vi "_System Polling.vi"   [LabVIEW 2012]
uses:
  <vilib>/rvi/DataTransferAndStorage/Container/Common/niFpgaContainerGetUniqueNameForEmu.vi
  <vilib>/rvi/Memory/Memory_Emulation/niFpgaMemoryEmulationCacheClearOnFirstRun.vi
  <vilib>/rvi/Memory/Memory_Emulation/nirvimemoryEmulationManagerCache_MakeExclusive.vi
  <vilib>/rvi/Memory/Memory_Emulation/niFpgaMemoryEmulationValidateCache.vi
  <vilib>/rvi/Memory/Memory_Emulation/nirvimemoryEmulationManagerCache_ReleaseExclusive.vi
  <vilib>/rvi/Memory/Memory_Emulation/nirvimemoryEmulationManagerCache_InsertValue.vi
  <vilib>/Utility/error.llb/Clear Errors.vi
  <vilib>/rvi/Emulation/niFpgaSctlEmulationGetInTimedLoop.vi
  <vilib>/rvi/Memory/Memory_Emulation/nirvimemoryEmulationManagerCache_GetValue.vi
  <vilib>/rvi/Memory/Memory_Emulation/nirvimemoryEmulationManagerCache_SetValue.vi
  <vilib>/rvi/Emulation/niFpgaSctlEmulationResourceMgr.vi
  <vilib>/rvi/DataTransferAndStorage/Container/XNode/niFpgaContainer.xnode
  <vilib>/rvi/Memory/Memory_Emulation/nirvimemoryEmulation.vi
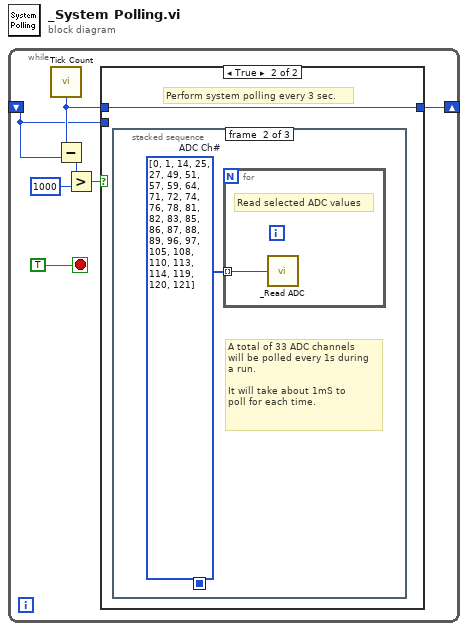
[diagram p0: block diagram]
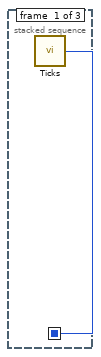
[diagram p3: hidden frame]
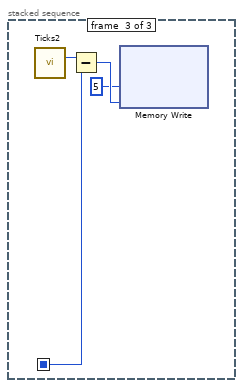
[diagram p4: hidden frame]
diagram:
  n1 = while {
    shift-right: [w1] -> _
    shift-left: _ -> [w2]
    stop <- TRUE stop-if-true
    n2 = call "Tick Count"() -> ("Tick Count(mSec)"=w3:u32)
    n3 = Subtract(x=w3, y=w2) -> (x-y=w6:u32)
    n4 = Greater?(x=w6, y=u32 1000) -> (0:w4:bool)
    n5 = case shown="True" w4 {
      tunnel: w3 -> [_ w9]
      tunnel: w2 -> [w8 _]
      tunnel: [w8 w9] -> w1
      frame False {
      }
      frame True {
        # "Perform system polling every 3 sec."
        n6 = stacked-sequence {
          seq-local: [w10 _ _] -> [_ _ w13]
          frame #0 {
            n7 = call "Ticks"() -> ("Tick Count(Ticks)"=w10:u16)
          }
          frame #1 {
            w11 = u8[] [0, 1, 14, 25, 27, 49, 51, 57, 59, 64, 71, 72, 74, 76, 78, 81, 82, 83, 85, 86, 87, 88, 89, 96, 97, 105, 108, 110, 113, 114, 119, 120, 121]  # ADC Ch#
            # "A total of 33 ADC channels\nwill be polled every 1s during\na run.\n\nIt will take about 1mS to\npoll for each time."
            n8 = for {
              tunnel: w11 -> [w12] mode=indexing
              # "Read selected ADC values"
              n9 = call "_Read ADC.vi"("Channel #"=w12) -> ()  [unwired: 1 out]
            }
          }
          frame #2 {
            n10 = call "Ticks2"() -> ("Tick Count(Ticks)"=w14:u16)
            n11 = Subtract(x=w14, y=w13) -> (x-y=w16:u16)
            n12 = xnode ("Memory Write")("Address"=u8 5, "Data"=w16) -> ()  [unwired: 1 in, 1 out]
          }
        }
      }
    }
  }
